vi "Local Antenna Method.vi"(11 "command":enum16{"connections", "reboot"}[](array[ring])) -> (3 "out":string[](array[string]))   [LabVIEW 2019]
uses:
  46b14fb0-980f-4cb7-b38b-6a9e02430269.vi
  <vilib>/JDP Science/JSONtext/Find Item.vi
  <vilib>/JDP Science/JSONtext/Next JSON Value.vi
  <vilib>/JDP Science/JSONtext/String Subset.vi
  <vilib>/JDP Science/JSONtext/Parsing/Advance past next JSON Value (inlined COPY).vi
  <vilib>/JDP Science/JSONtext/Parsing/Advance past whitespace.vi
  <vilib>/JDP Science/JSONtext/Parsing/Advance past String.vi
  <vilib>/JDP Science/JSONtext/Parsing/Advance past Number.vi
  <vilib>/JDP Science/JSONtext/Parsing/Advance past Line Ending.vi
  <vilib>/JDP Science/JSONtext/Parsing/Parse Full Path or Item Name.vi
  <vilib>/JDP Science/JSONtext/Parsing/Advance past Array.vi
  <vilib>/JDP Science/JSONtext/Parsing/Advance past Object.vi
  <vilib>/JDP Science/JSONtext/support/Error Cluster From Code.vi
  <vilib>/JDP Science/JSONtext/Offset/Find Item Locations by Path.vi
  <vilib>/JDP Science/JSONtext/JSON text to Variant.vi
  <vilib>/JDP Science/JSONtext/LVClass Serializer/JSONtext LVClass Serializer.lvclass
panel:
  in  "patch reboot":string="curl -X 'PATCH' 'http://%s/api/v1/system' -H 'accept: */*' -H 'Authorization: Bearer %s' -H 'Content-Type: application/json' -d '{ \"reboot\": true }'"
  in  "get connections":string="curl -X 'GET' 'http://%s/api/v1/wlan/interfaces/1/connections' -H 'accept: */*' -H 'Authorization: Bearer %s' -H 'Content-Type: ' -d ''"
  in  "revoke token":string="curl -X 'POST' 'http://%s/auth/revoke' -H 'accept: */*' -H 'Authorization: Bearer %s' -H 'Content-Type: application/x-www-form-urlencoded' -d 'token=%s'"
  in  "get token":string="curl -X 'POST' 'http://%s/auth/token' -H 'accept: */*' -H 'Authorization: Basic %s' -H 'Content-Type: application/x-www-form-urlencoded' -d 'grant_type=client_credentials'"
  out "token":string
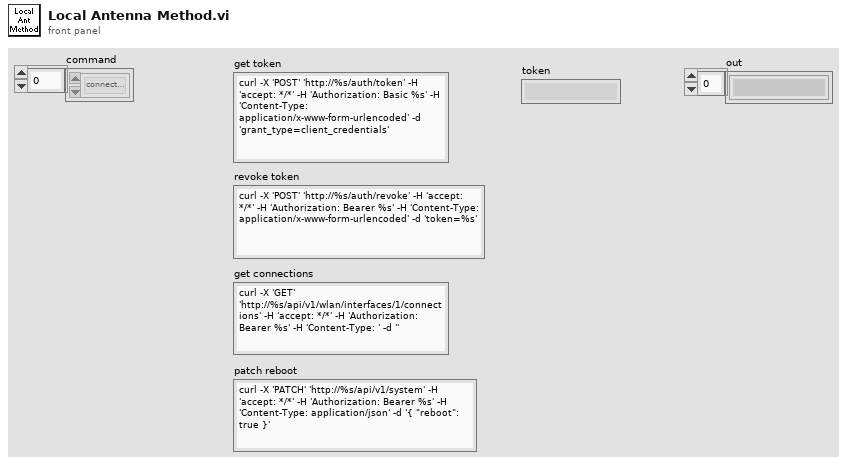
[diagram p1: front panel]
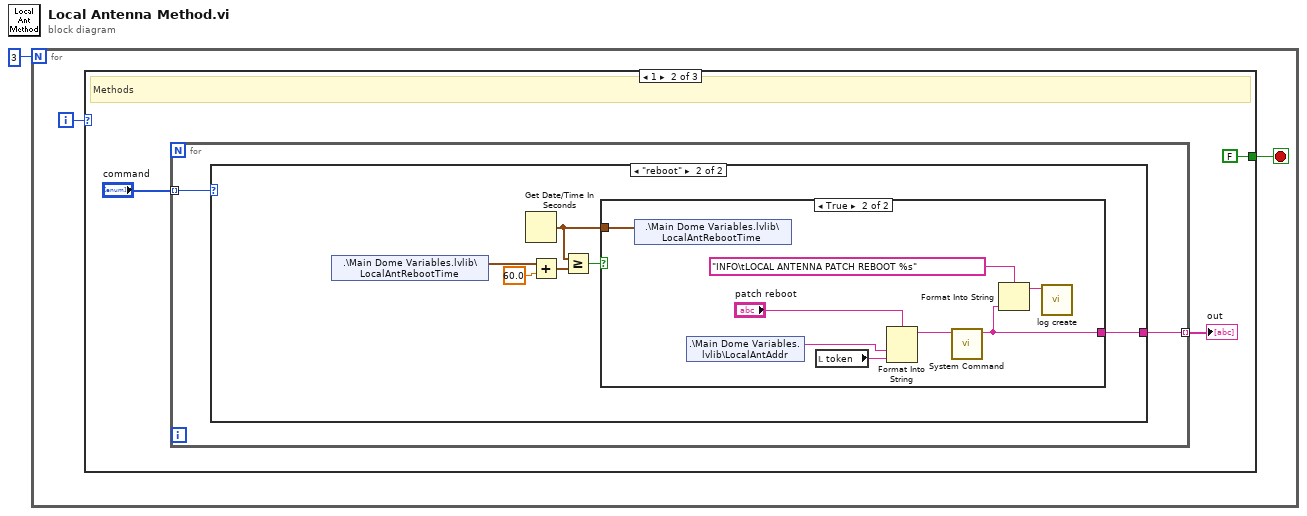
[diagram p0: block diagram]
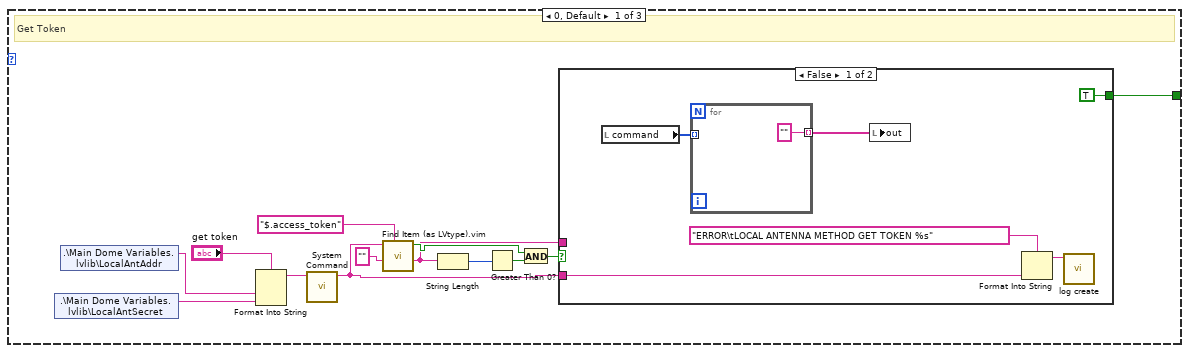
[diagram p2: hidden frame]
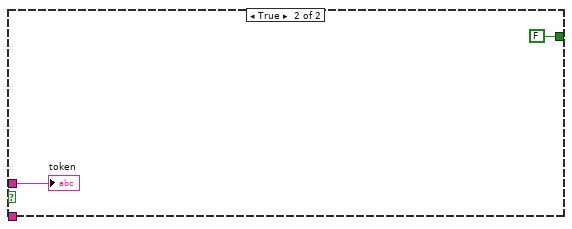
[diagram p3: hidden frame]
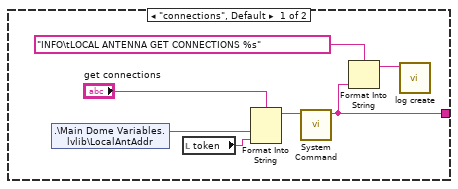
[diagram p4: hidden frame]
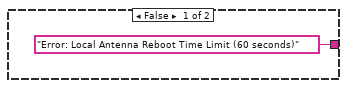
[diagram p5: hidden frame]
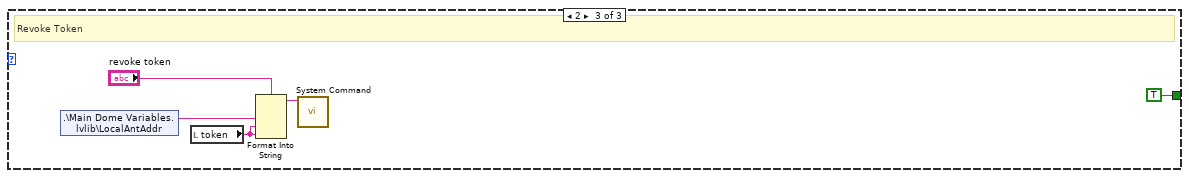
[diagram p6: hidden frame]
diagram:
  n1 = for {
    N: 3 -> [_]
    i -> [w3]
    stop <- w2 stop-if-true
    n2 = case shown="1" w3 {
      tunnel: [w9 FALSE TRUE] -> w2
      frame 0, Default {
        # "Get Token"
        n3 = shared-variable ".\\Main Dome Variables.lvlib\\LocalAntSecret"() -> (w15:string)  [unwired: 1 in, 1 out]
        n4 = shared-variable ".\\Main Dome Variables.lvlib\\LocalAntAddr"() -> (w14:string)  [unwired: 1 in, 1 out]
        n5 = Format Into String(format string="get token", w14, w15) -> (resulting string=w16:string)  [unwired: 2 in, 1 out]
        n6 = call "System Command.vi"("command"=w16) -> ("standard output"=w10:string)  [unwired: 7 in, 3 out]
        n7 = call "Find Item (as LVtype).vim"("$Path or Item Name"="$.access_token", "Data Type and Default Value"="", "JSON"=w10) -> ("Data"=w6:string, "Found"=w7:bool)  [unwired: 5 in, 2 out]
        n8 = String Length(string=w6) -> (length=w5:i32)
        n9 = Greater Than 0?(x=w5) -> (x > 0?=w4:bool)
        n10 = And(x=w7, y=w4) -> (x .and. y?=w8:bool)
        n11 = case shown="False" w8 {
          tunnel: w6 -> [_ w25]
          tunnel: w10 -> [w21 _]
          tunnel: [TRUE FALSE] -> w9
          frame False {
            n12 = local read "command"() -> (w18:enum16{"connections", "reboot"}[])
            n13 = for {
              tunnel: w18 -> [_] mode=indexing
              tunnel: [""] -> w17 mode=indexing
            }
            n14 = local write "out"(w17) -> ()
            n15 = Format Into String(format string="ERROR\tLOCAL ANTENNA METHOD GET TOKEN %s", w21) -> (resulting string=w20:string)  [unwired: 2 in, 1 out]
            n16 = call "log create.vi"("message"=w20) -> ()  [unwired: 11 in]
          }
          frame True {
            "token" <- w25
          }
        }
      }
      frame 1 {
        # "Methods"
        n17 = for {
          tunnel: "command" -> [w30] mode=indexing
          tunnel: [w29] -> w26 mode=indexing
          n18 = case shown="\"reboot\"" w30 {
            tunnel: [w33 w43] -> w29
            frame "connections", Default {
              n19 = shared-variable ".\\Main Dome Variables.lvlib\\LocalAntAddr"() -> (w36:string)  [unwired: 1 in, 1 out]
              n20 = local read "token"() -> (w35:string)
              n21 = Format Into String(format string="get connections", w36, w35) -> (resulting string=w34:string)  [unwired: 2 in, 1 out]
              n22 = call "System Command.vi"("command"=w34) -> ("standard output"=w33:string)  [unwired: 7 in, 3 out]
              n23 = Format Into String(format string="INFO\tLOCAL ANTENNA GET CONNECTIONS %s", w33) -> (resulting string=w31:string)  [unwired: 2 in, 1 out]
              n24 = call "log create.vi"("message"=w31) -> ()  [unwired: 11 in]
            }
            frame "reboot" {
              n25 = shared-variable ".\\Main Dome Variables.lvlib\\LocalAntRebootTime"() -> (w41:timestamp)  [unwired: 1 in, 1 out]
              n26 = Get Date/Time In Seconds() -> (seconds since 1Jan1904=w38:timestamp)
              n27 = Add(x=w41, y=60.0) -> (x+y=w40:timestamp)
              n28 = Greater Or Equal?(x=w38, y=w40) -> (x >= y?=w39:bool)
              n29 = case shown="True" w39 {
                tunnel: ["Error: Local Antenna Reboot Time Limit (60 seconds)" ("standard output") w48] -> w43
                tunnel: w38 -> [_ w46]
                frame False {
                }
                frame True {
                  n30 = shared-variable ".\\Main Dome Variables.lvlib\\LocalAntRebootTime"(w46) -> ()  [unwired: 1 in, 1 out]
                  n31 = shared-variable ".\\Main Dome Variables.lvlib\\LocalAntAddr"() -> (w51:string)  [unwired: 1 in, 1 out]
                  n32 = local read "token"() -> (w50:string)
                  n33 = Format Into String(format string="patch reboot", w51, w50) -> (resulting string=w49:string)  [unwired: 2 in, 1 out]
                  n34 = call "System Command.vi"("command"=w49) -> ("standard output"=w48:string)  [unwired: 7 in, 3 out]
                  n35 = Format Into String(format string="INFO\tLOCAL ANTENNA PATCH REBOOT %s", w48) -> (resulting string=w45:string)  [unwired: 2 in, 1 out]
                  n36 = call "log create.vi"("message"=w45) -> ()  [unwired: 11 in]
                }
              }
            }
          }
        }
        "out" <- w26
      }
      frame 2 {
        # "Revoke Token"
        n37 = shared-variable ".\\Main Dome Variables.lvlib\\LocalAntAddr"() -> (w55:string)  [unwired: 1 in, 1 out]
        n38 = local read "token"() -> (w54:string)
        n39 = Format Into String(format string="revoke token", w55, w54, w54) -> (resulting string=w57:string)  [unwired: 2 in, 1 out]
        n40 = call "System Command.vi"("command"=w57) -> ()  [unwired: 7 in, 4 out]
      }
    }
  }
